vi "Variables a enviar WEB.vi"(6 "#Variables":enum16{"1 Variable", "Mas de una Variable"}(ring), 8 "error in":errorcluster, 10 "Array Data":dbl[](array[numeric]), 11 "Nombre Variable":string) -> (0 "error out":errorcluster, 3 "Trama Json":string)   [LabVIEW 2020, in "Client HTTP POST.lvlib"]
uses:
  Client HTTP POST.lvlib
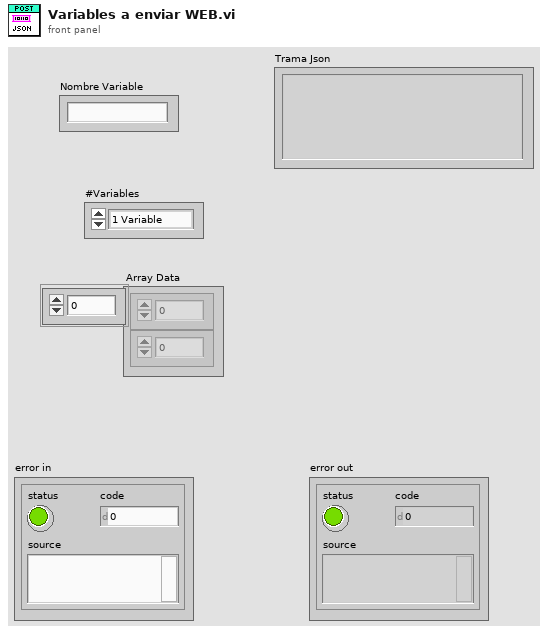
[diagram p1: front panel]
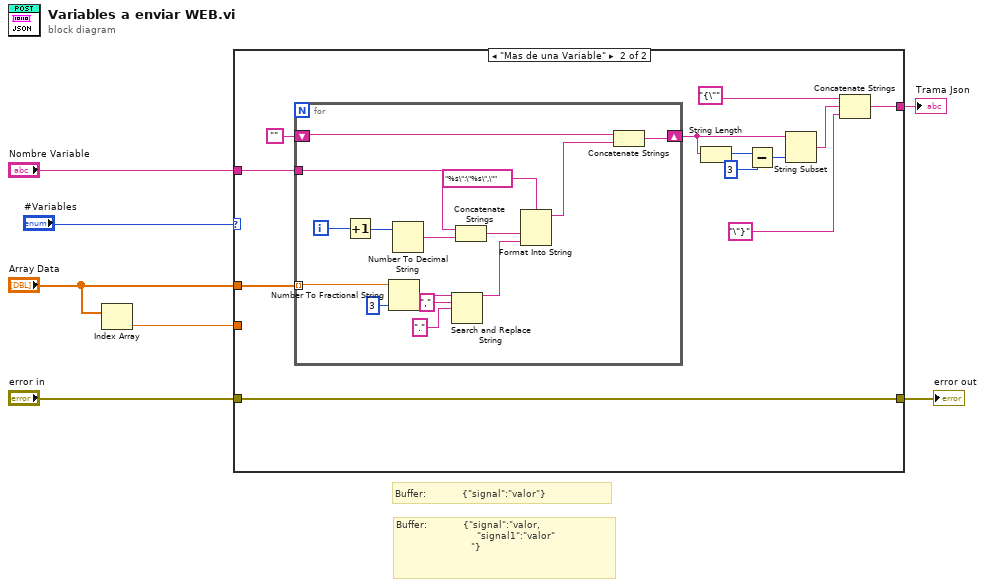
[diagram p0: block diagram]
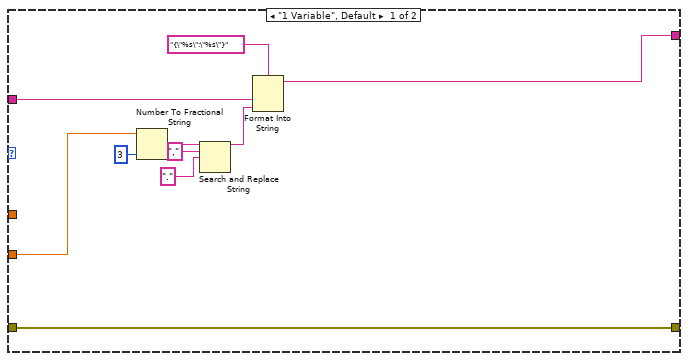
[diagram p2: hidden frame]
diagram:
  # "Buffer:            {\"signal\":\"valor,\n                           \"signal1\":\"valor\"\n                         \"}"
  # "Buffer:            {\"signal\":\"valor\"}"
  n1 = Index Array(array="Array Data") -> (element=w2:dbl)  [unwired: 1 in]
  n2 = case shown="\"Mas de una Variable\"" "#Variables" {
    tunnel: "Array Data" -> [_ w29]
    tunnel: "Nombre Variable" -> [w11 w28]
    tunnel: [w10 w19] -> w6
    tunnel: [w9 w18] -> w5
    tunnel: "error in" -> [w9 w18]
    tunnel: w2 -> [w8 _]
    frame "1 Variable", Default {
      n3 = Number To Fractional String(number=w8, precision (6)=i16 3) -> (F-format string=w16:string)  [unwired: 2 in]
      n4 = Search and Replace String(input string=w16, search string=",", replace string="." ("replace string (\"\")")) -> (result string=w17:string)  [unwired: 5 in, 3 out]
      n5 = Format Into String(format string="{\"%s\":\"%s\"}", w11, w17) -> (resulting string=w10:string)  [unwired: 2 in, 1 out]
    }
    frame "Mas de una Variable" {
      n6 = for {
        tunnel: w29 -> [w44] mode=indexing
        shift-right: [w35] -> w26
        shift-left: "" -> [w37]
        tunnel: w28 -> [w33]
        i -> [w39]
        n7 = Increment(x=w39) -> (x+1=w34:i32)
        n8 = Number To Fractional String(number=w44, precision (6)=i16 3) -> (F-format string=w42:string)  [unwired: 2 in]
        n9 = Number To Decimal String(number=w34) -> (decimal integer string=w32:string)  [unwired: 1 in]
        n10 = Search and Replace String(input string=w42, search string=",", replace string="." ("replace string (\"\")")) -> (result string=w30:string)  [unwired: 5 in, 3 out]
        n11 = Concatenate Strings(w33, w32) -> (w31:string)
        n12 = Format Into String(format string="%s\":\"%s\",\"", w31, w30) -> (resulting string=w36:string)  [unwired: 2 in, 1 out]
        n13 = Concatenate Strings(w37, w36) -> (w35:string)
      }
      n14 = String Length(string=w26) -> (length=w22:i32)
      n15 = Subtract(x=w22, y=3) -> (x-y=w20:i32)
      n16 = String Subset(string=w26, length (rest)=w20) -> (substring=w24:string)  [unwired: 1 in]
      n17 = Concatenate Strings("{\"" ("format string"), w24, "\"}" ("format string")) -> (w19:string)
    }
  }
  "Trama Json" <- w6
  "error out" <- w5
